vi "SaveDataDigitizerV1729.vi"(4 "Module":string="Digitizer Data", 5 "Save Data?":bool, 6 "File Handle":T1 format="%.0x", 7 "# Samples after Trig":u16, 8 "error in (no error)":errorcluster, 9 "String":string, 10 "Digitizer Waveforms":u32[](array[numeric]), 11 "Digitizer TRIG_REC":u32) -> (0 "error out":errorcluster, 1 "File Handle Out":T1 format="%.0x", 2 "Channel Data":u16[][](array[numeric]))   [LabVIEW 2014]
uses:
  <vilib>/addons/h5labview2/base/hid_t.ctl
  <vilib>/addons/h5labview2/base/lib_path.vi
  <vilib>/addons/h5labview2/base/H5Equery.vi
  <vilib>/addons/h5labview2/dataset/H5Dwrite.llb/H5Dwrite.xnode
  <vilib>/addons/h5labview2/group/H5G.lvlib
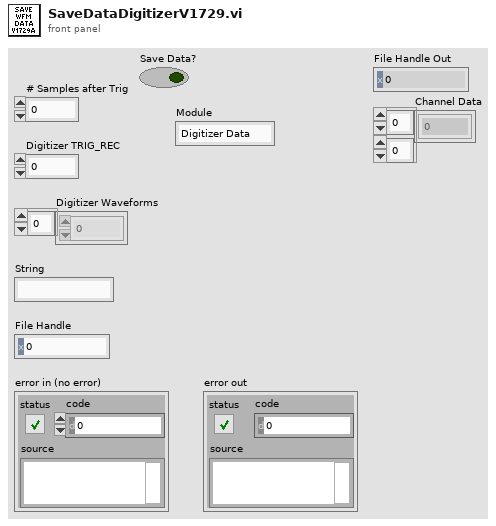
[diagram p1: front panel]
types:
  T1 = typedef "hid_t.ctl" = i32
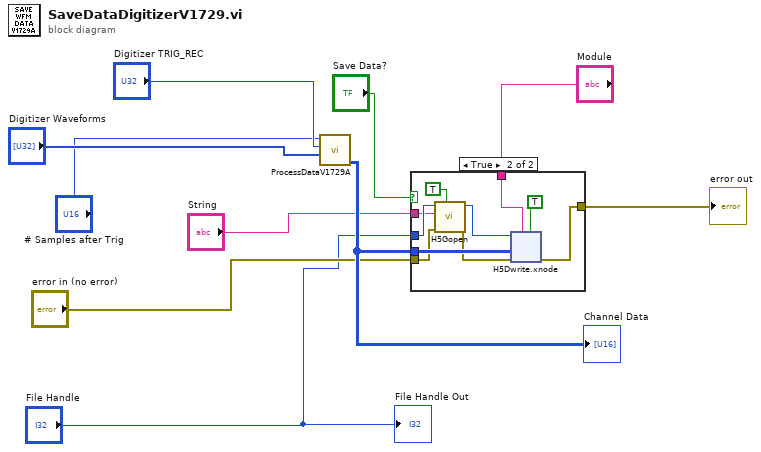
[diagram p0: block diagram]
diagram:
  n1 = call "ProcessDataV1729A.vi"("Buffer"="Digitizer Waveforms", "TRIG_REC"="Digitizer TRIG_REC", "# Samples after Trig"="# Samples after Trig") -> ("Channel Data"=w5:u16[][])  [unwired: 7 in, 1 out]
  "Channel Data" <- w5
  n2 = case shown="True" "Save Data?" {
    tunnel: "error in (no error)" -> [w11 w15]
    tunnel: "File Handle" -> [_ w14]
    tunnel: [w11 w20] -> w8
    tunnel: "Module" -> [_ w19]
    tunnel: w5 -> [_ w18]
    tunnel: "String" -> [_ w13]
    frame False {
    }
    frame True {
      n3 = call <vilib>:"H5Gopen.vi"("create? (F)"=TRUE, "error in (no error)"=w15, "name"=w13, "ref in"=w14) -> ("error out"=w16:errorcluster, "group out"=w17:T1)  [unwired: 6 in]
      n4 = xnode "H5Dwrite.xnode"("replace? (F)"=TRUE, "dataset name"=w19, "error in (no error)"=w16, "data"=w18, "ref in"=w17) -> ("error out"=w20:errorcluster)  [unwired: 2 in, 2 out]
    }
  }
  "error out" <- w8
  "File Handle Out" <- "File Handle"
